vi "WT-Velocity+Density.vi"() -> ()   [LabVIEW 2017]
uses:
  <vilib>/Analysis/baseanly.llb/Mean (DBL).vi
  Globals/mainWTControl.vi
  <vilib>/Analysis/NI_AALBase.lvlib
panel:
  in  "Delay Time (s)":dbl=1.0
  out "mean 2":dbl format="%0.3f"
  out "mean":dbl format="%0.3f"
  out "Density":dbl[](graph)
  out "Velocity":dbl[](graph)
  in  "stop":bool
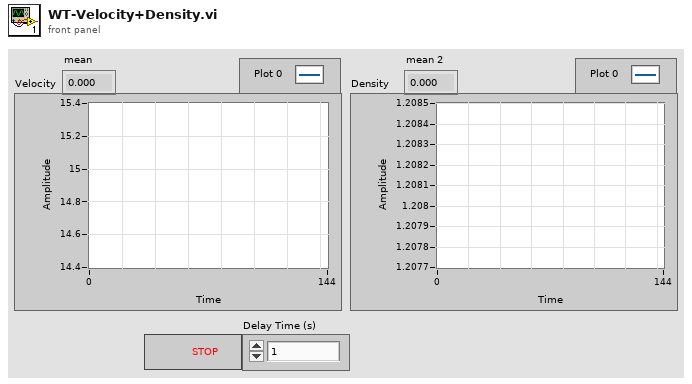
[diagram p1: front panel]
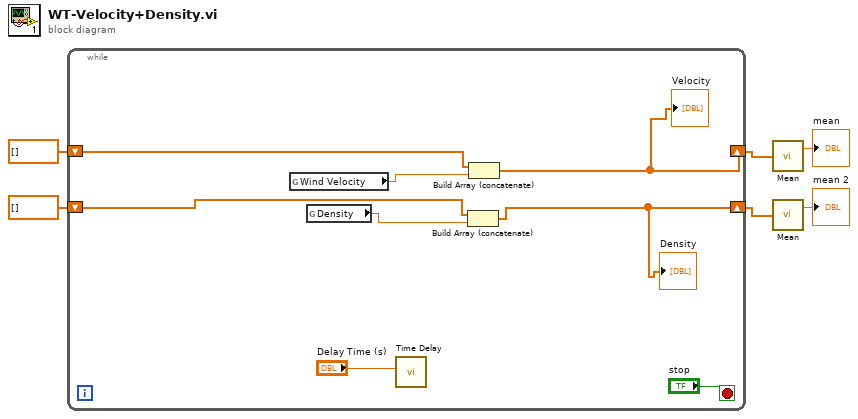
[diagram p0: block diagram]
diagram:
  n1 = while {
    shift-right: [w8] -> w3
    shift-left: dbl[] [] -> [w10]
    shift-right: [w9] -> w4
    shift-left: dbl[] [] -> [w11]
    stop <- "stop" stop-if-true
    n2 = global read "mainWTControl.vi" "Wind Velocity"() -> (w12:dbl)
    n3 = global read "mainWTControl.vi" "Density"() -> (w13:dbl)
    n4 = call "Time Delay"("Delay Time (s)"="Delay Time (s)") -> ()  [unwired: 10 in, 1 out]
    n5 = Build Array (concatenate)(w10, w13) -> (w8:dbl[])
    "Density" <- w8
    n6 = Build Array (concatenate)(w11, w12) -> (w9:dbl[])
    "Velocity" <- w9
  }
  n7 = call-poly <vilib>:"Mean.vi"("X"=w4) -> ("mean"=→"mean":dbl)  [unwired: 1 out]
  n8 = call-poly <vilib>:"Mean.vi"("X"=w3) -> ("mean"=→"mean 2":dbl)  [unwired: 1 out]
